vi "proba_2.vi"() -> ()   [LabVIEW 2015]
uses:
  <vilib>/MakerHub/LINX/Public/Peripherals/Digital/Digital Write N Chans.vi
  <vilib>/MakerHub/LINX/Public/Peripherals/Analog/Analog Read 1 Chan.vi
  <vilib>/MakerHub/LINX/Private/Local IO/LinxDigitalWrite.vi
  <vilib>/MakerHub/LINX/Public/Utilities/Check Channel.vi
  <vilib>/MakerHub/LINX/Public/Peripherals/Analog/Analog Read N Chans.vi
  <vilib>/MakerHub/LINX/Private/Local IO/LinxAnalogRead.vi
  <vilib>/MakerHub/LINX/Public/Utilities/Open Serial.vi
  <vilib>/MakerHub/LINX/Private/Utilties/Generate Error.vi
  <vilib>/MakerHub/LINX/LMH-LINX.lvlib
panel:
  out "x-y":u32
  out "appended array":bool[](array[boolean])
  in  "Stop Button":bool
  in  "Sample_1 (time)":dbl[][](array[numeric])
  in  "stop":bool
  in  "Sample_2 (time)":dbl[][](array[numeric])
  in  "Sample_3 (time)":dbl[][](array[numeric])
  in  "Sample_4 (time)":dbl[][](array[numeric])
  in  "LED_5 (time)":dbl[][](array[numeric])
  in  "Temp/Gap_1 (time)":dbl[][](array[numeric])
  in  "Temp/Gap_2 (time)":dbl[][](array[numeric])
  in  "Temp/Gap_3 (time)":dbl[][](array[numeric])
  in  "Temp/Gap_4 (time) 2":dbl[][](array[numeric])
  out "Ref":dbl(graph)
  in  "LED":refnum<visa-resource-name>="N/A"
  out "3":dbl(graph)
  out "2":dbl(graph)
  out "4":dbl(graph)
  out "1":dbl(graph)
  in  "milliseconds to wait":u32
  in  "Serial Port Analog":refnum<visa-resource-name>="N/A"
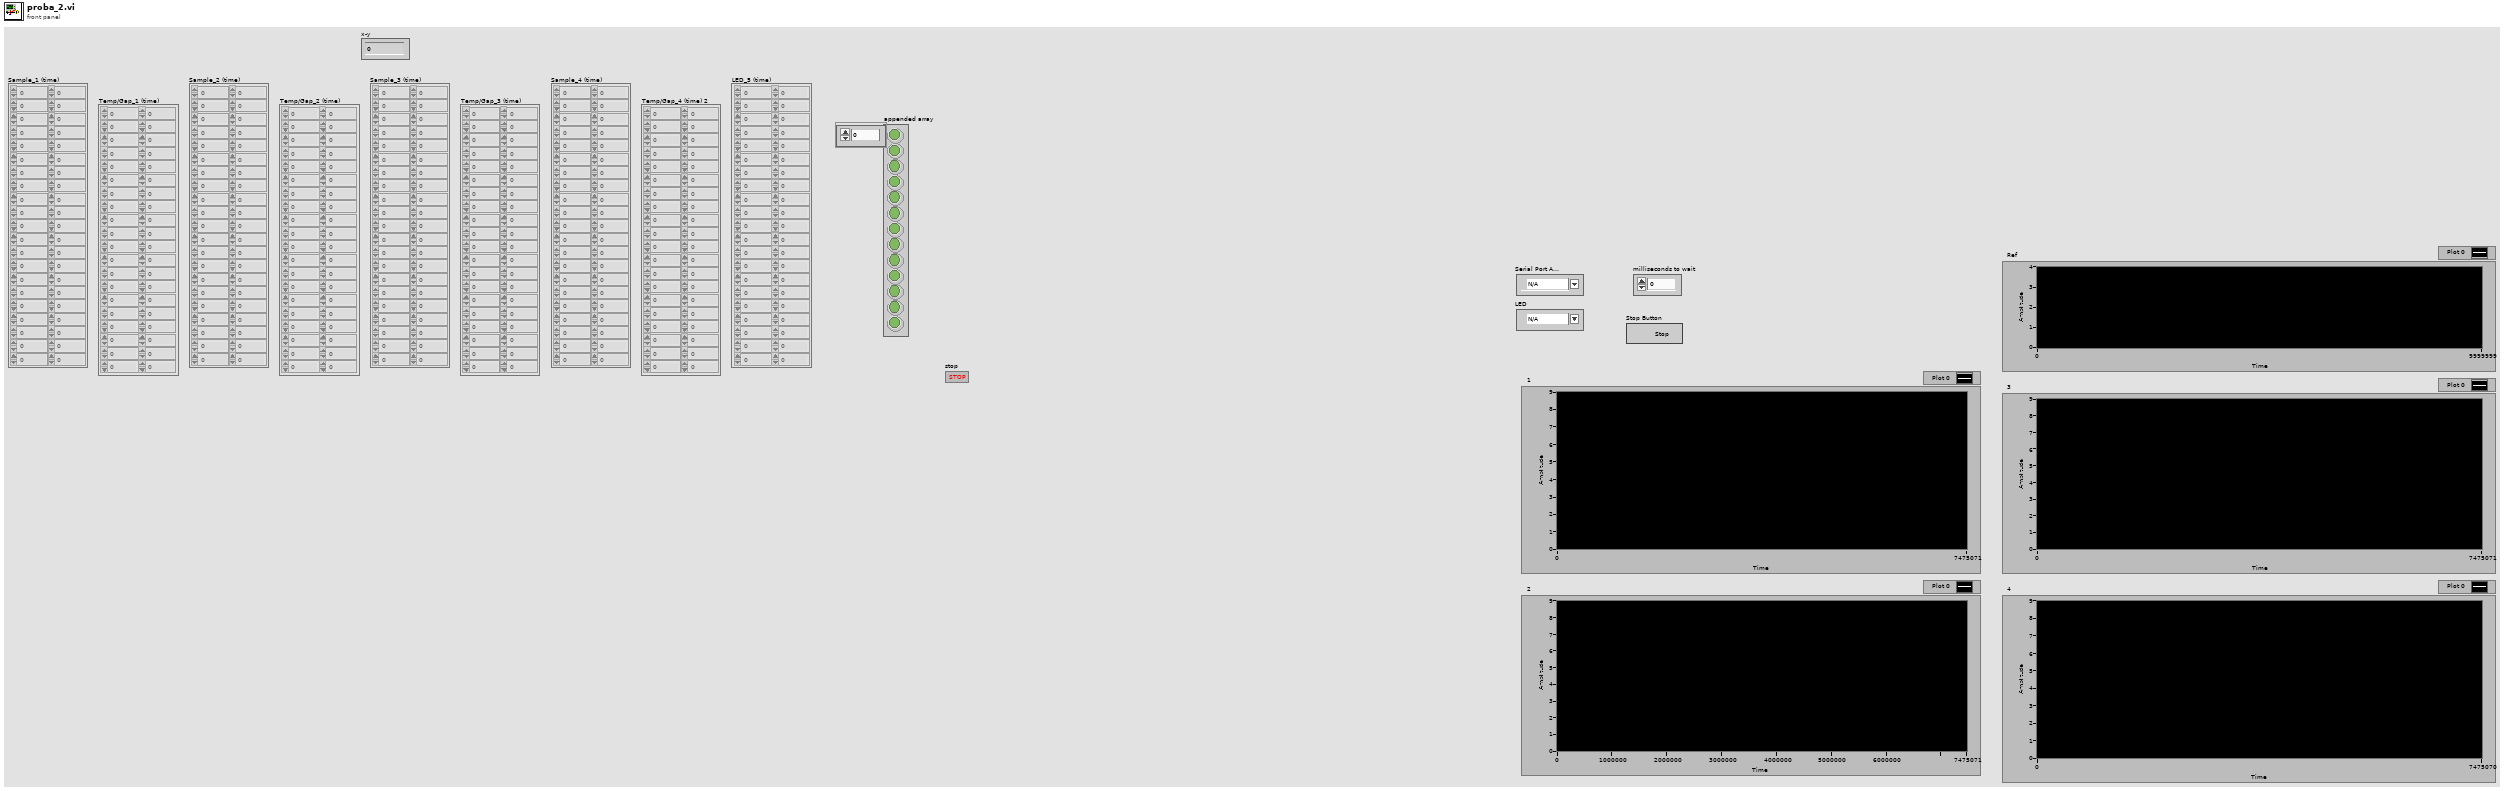
[diagram p1: front panel]
types:
  T1 = enum16{"open", "replace", "create", "open or create", "replace or create", "replace or create with confirmation"}
  T2 = typedef "LMH-LINX.lvlib/LINX Ref.ctl" = cluster{"IO":T3, "Interface":T4, "LINX Device Config":T5}
  T3 = typedef "LMH-LINX.lvlib/Platform.ctl" = enum16{"Remote", "Local"}
  T4 = typedef "LMH-LINX.lvlib/Interface.ctl" = enum16{"Serial", "TCP"}
  T5 = typedef "LMH-LINX.lvlib/Device.lvlib/LINX Device Config.ctl" = cluster{"Interface":T4, "COM Port":refnum<visa-resource-name>, "TCP Configuration":T6, "Device Family":u8, "Device ID":u8, "Device Name":string, "TCP Ref":refnum<k5>, "Channels":T7}
  T6 = typedef "LMH-LINX.lvlib/Device.lvlib/TCP Config.ctl" = cluster{"IP Address":string, "Port":u16}
  T7 = typedef "LMH-LINX.lvlib/Channels.ctl" = cluster{"DI":u8[], "DO":u8[], "AI":u8[], "AO":u8[], "PWM":u8[], "QE":u8[], "UART":u8[], "I2C 2":u8[], "SPI":u8[], "CAN":u8[], "Servo":u8[], "AI Ref (V)":dbl, "AI Resolution (Bits)":u8, "AO Ref (V)":dbl, "AO Resolution (Bits)":u8}
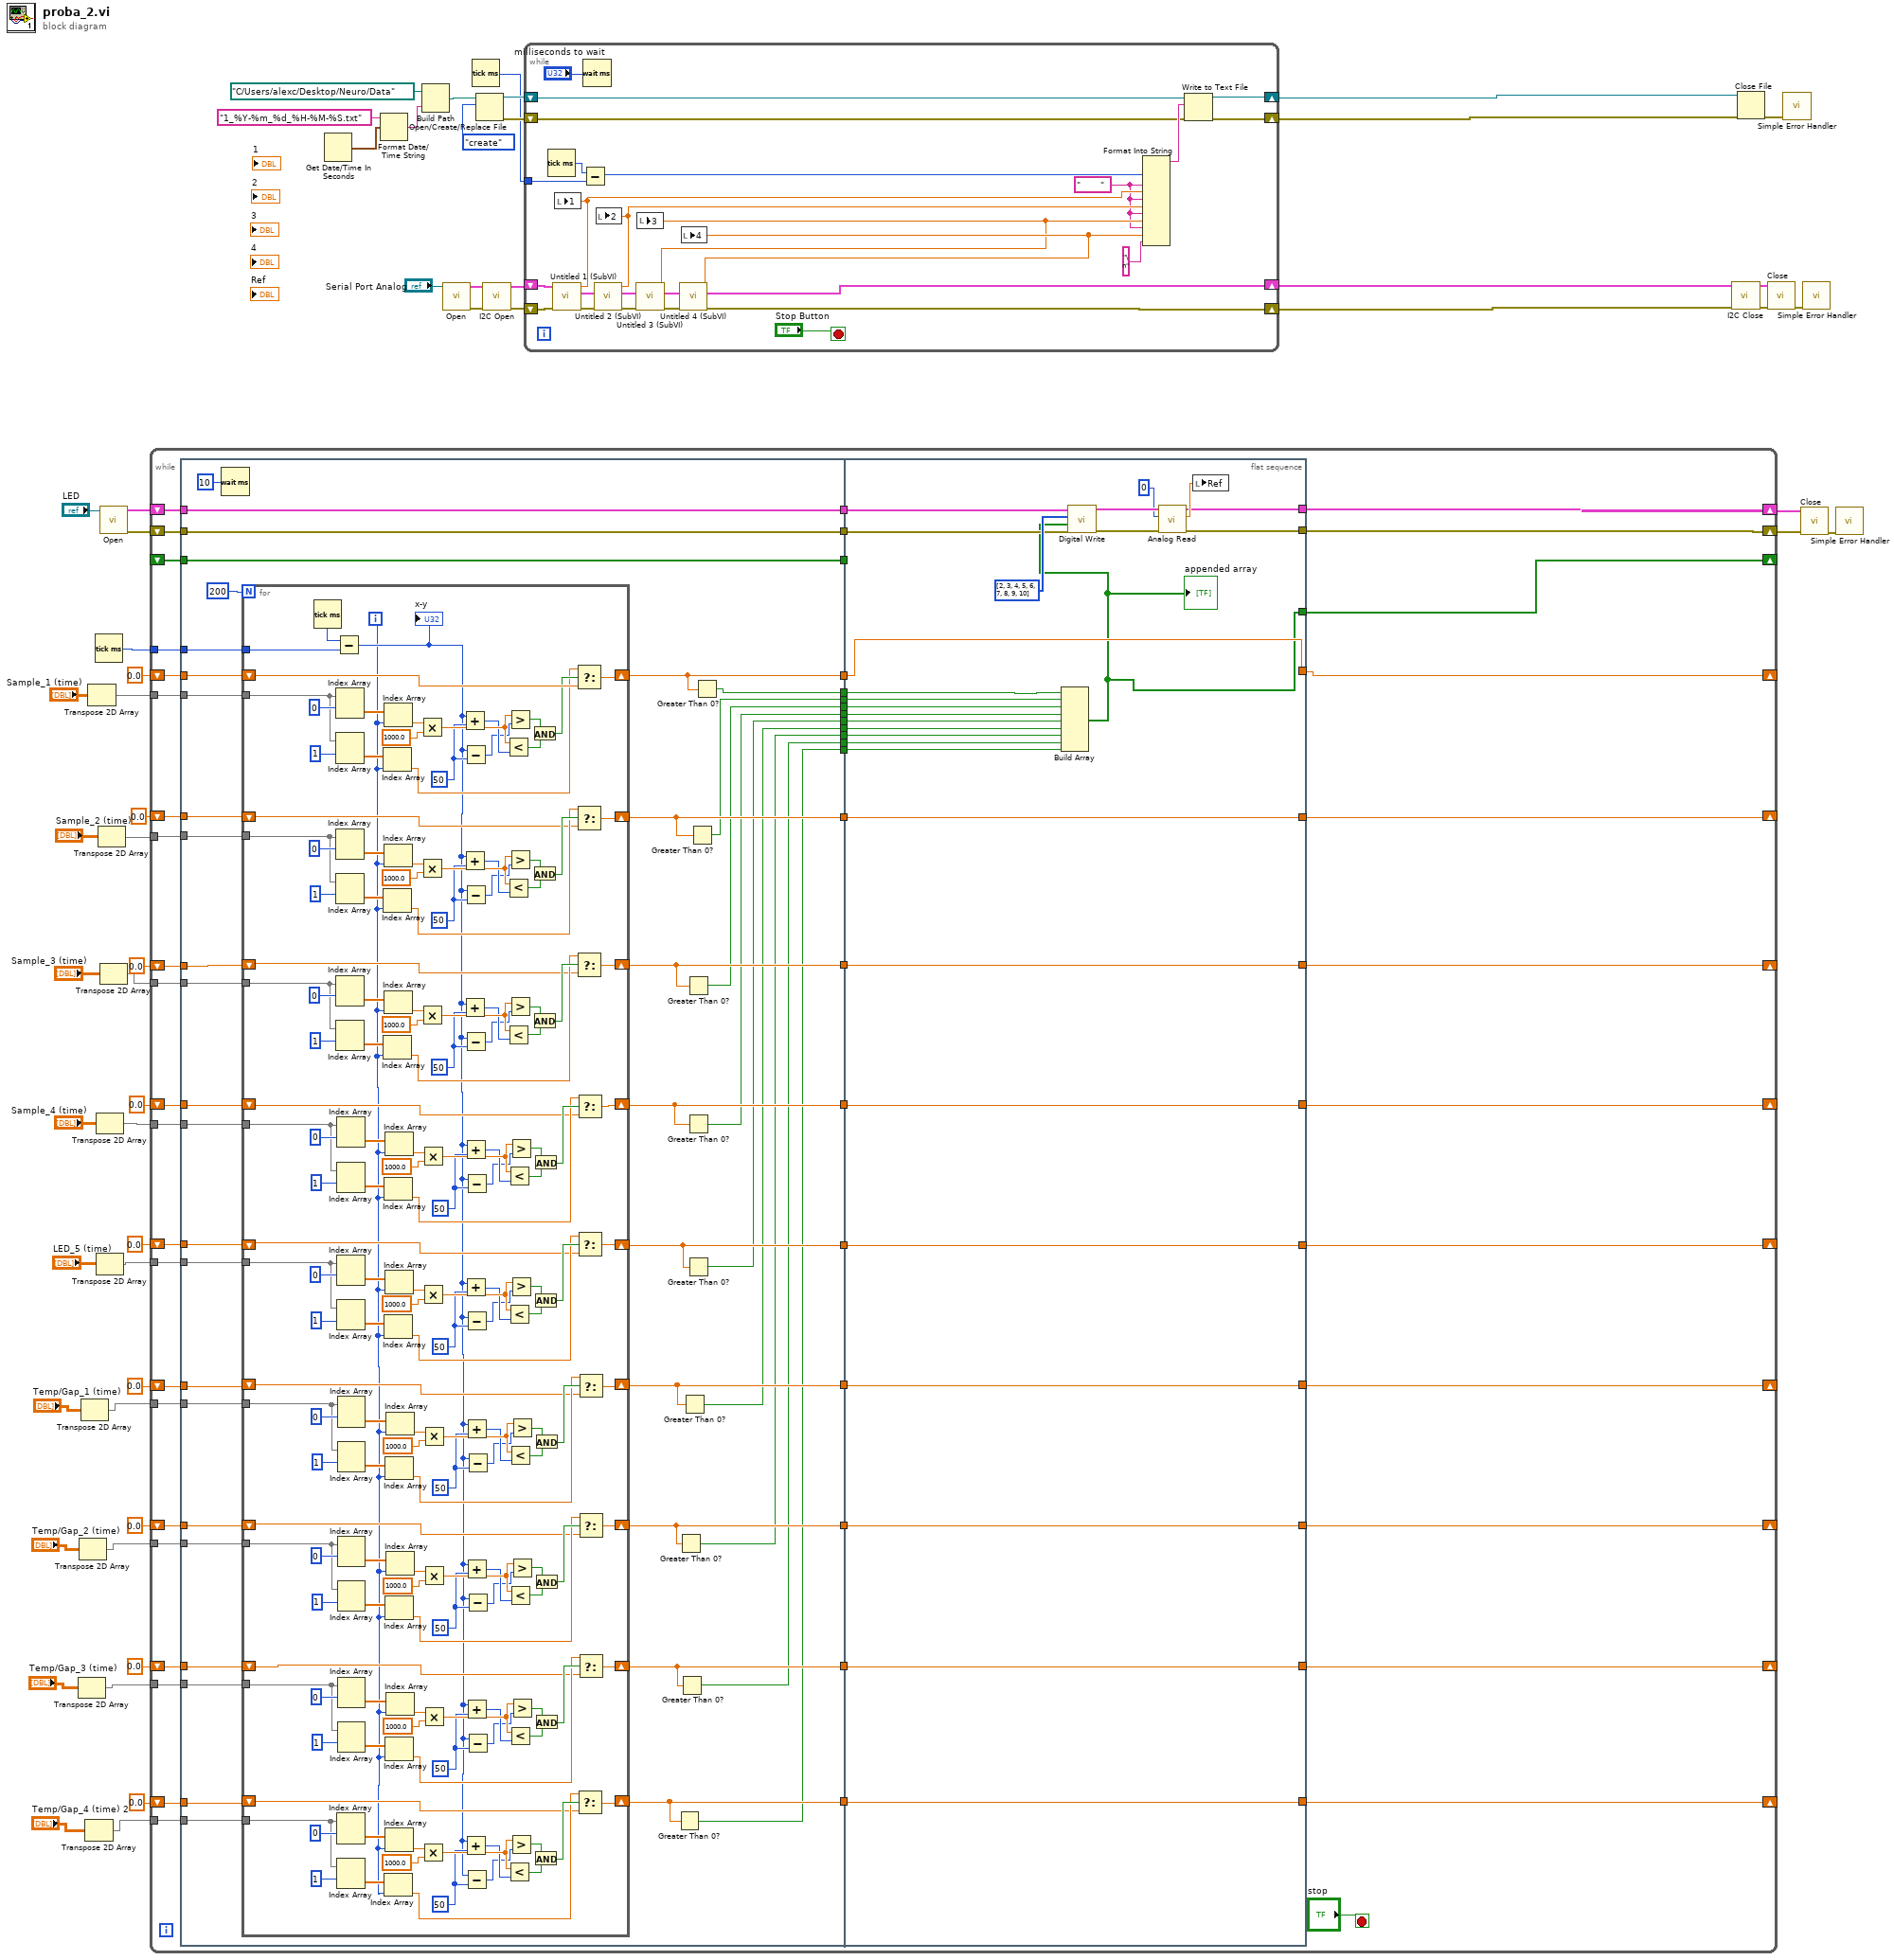
[diagram p0: block diagram]
diagram:
  n1 = Transpose 2D Array(2D array="Temp/Gap_3 (time)") -> (transposed array=w11:dbl[][])
  n2 = Transpose 2D Array(2D array="Temp/Gap_2 (time)") -> (transposed array=w12:dbl[][])
  n3 = Transpose 2D Array(2D array="Temp/Gap_1 (time)") -> (transposed array=w13:dbl[][])
  n4 = Transpose 2D Array(2D array="Temp/Gap_4 (time) 2") -> (transposed array=w10:dbl[][])
  n5 = Transpose 2D Array(2D array="Sample_1 (time)") -> (transposed array=w26:dbl[][])
  n6 = Tick Count (ms)() -> (millisecond timer value=w30:u32)
  n7 = Transpose 2D Array(2D array="Sample_4 (time)") -> (transposed array=w15:dbl[][])
  n8 = Transpose 2D Array(2D array="LED_5 (time)") -> (transposed array=w14:dbl[][])
  n9 = Transpose 2D Array(2D array="Sample_2 (time)") -> (transposed array=w24:dbl[][])
  n10 = call-poly <vilib>:"Open.vi"("Serial Port"="LED") -> ("Error Out"=w31:errorcluster, "LINX Resource"=w32:T2)  [unwired: 8 in, 1 out]
  n11 = Transpose 2D Array(2D array="Sample_3 (time)") -> (transposed array=w16:dbl[][])
  n12 = while {
    tunnel: w30 -> [w110]
    shift-right: [w60] -> _
    shift-left: 0.0 ("Numeric") -> [w112]
    shift-right: [w66] -> w29
    shift-left: w32 -> [w63]
    shift-right: [w65] -> w28
    shift-left: w31 -> [w61]
    tunnel: w26 -> [w109]
    tunnel: w24 -> [w108]
    shift-right: [w85] -> _
    shift-left: 0.0 ("Numeric") -> [w107]
    tunnel: w11 -> [w106]
    tunnel: w16 -> [w105]
    tunnel: w15 -> [w104]
    tunnel: w14 -> [w103]
    tunnel: w13 -> [w102]
    tunnel: w12 -> [w101]
    tunnel: w10 -> [w100]
    shift-right: [w86] -> _
    shift-left: 0.0 ("Numeric") -> [w99]
    shift-right: [w87] -> _
    shift-left: 0.0 ("Numeric") -> [w98]
    shift-right: [w88] -> _
    shift-left: 0.0 ("Numeric") -> [w97]
    shift-right: [w90] -> _
    shift-left: 0.0 ("Numeric") -> [w96]
    shift-right: [w91] -> _
    shift-left: 0.0 ("Numeric") -> [w95]
    shift-right: [w92] -> _
    shift-left: 0.0 ("Numeric") -> [w94]
    shift-right: [w89] -> _
    shift-left: 0.0 ("Numeric") -> [w93]
    shift-right: [w59] -> _
    shift-left: _ -> [w58]
    stop <- "stop" stop-if-true
    n13 = flat-sequence {
      tunnel: w112 -> [w154]
      tunnel: w110 -> [w153]
      tunnel: w109 -> [w152]
      tunnel: w108 -> [w149]
      tunnel: w107 -> [w148]
      tunnel: w106 -> [w147]
      tunnel: w105 -> [w146]
      tunnel: w104 -> [w145]
      tunnel: w103 -> [w144]
      tunnel: w102 -> [w143]
      tunnel: w101 -> [w142]
      tunnel: w100 -> [w141]
      tunnel: w99 -> [w140]
      tunnel: w98 -> [w139]
      tunnel: w97 -> [w138]
      tunnel: w96 -> [w137]
      tunnel: w95 -> [w136]
      tunnel: w94 -> [w135]
      tunnel: w93 -> [w134]
      tunnel: [w133] -> w84
      tunnel: [w132] -> w83
      tunnel: [w131] -> w82
      tunnel: [w130] -> w81
      tunnel: [w129] -> w80
      tunnel: [w128] -> w79
      tunnel: [w127] -> w78
      tunnel: [w126] -> w77
      tunnel: [w125] -> w76
      tunnel: [w124] -> w75
      tunnel: [w123] -> w74
      tunnel: [w122] -> w73
      tunnel: [w121] -> w72
      tunnel: [w120] -> w71
      tunnel: [w119] -> w70
      tunnel: [w118] -> w69
      tunnel: [w117] -> w68
      tunnel: [w116] -> w67
      tunnel: [w115] -> w64
      tunnel: w63 -> [w115]
      tunnel: [w114] -> w62
      tunnel: w61 -> [w114]
      tunnel: w58 -> [w113]
      tunnel: [w113] -> w57
      tunnel: [w332] -> w85
      tunnel: [w333] -> w86
      tunnel: [w334] -> w87
      tunnel: [w335] -> w88
      tunnel: [w336] -> w89
      tunnel: [w337] -> w90
      tunnel: [w338] -> w91
      tunnel: [w339] -> w92
      tunnel: w84 -> [w339]
      tunnel: w83 -> [w338]
      tunnel: w82 -> [w337]
      tunnel: w81 -> [w336]
      tunnel: w80 -> [w335]
      tunnel: w79 -> [w334]
      tunnel: w78 -> [w333]
      tunnel: w77 -> [w332]
      tunnel: w76 -> [w326]
      tunnel: w75 -> [w322]
      tunnel: w74 -> [w321]
      tunnel: w73 -> [w320]
      tunnel: w72 -> [w319]
      tunnel: w71 -> [w318]
      tunnel: w70 -> [w317]
      tunnel: w69 -> [w316]
      tunnel: w68 -> [w315]
      tunnel: w67 -> [w325]
      tunnel: [w326] -> w60
      tunnel: [w324] -> w66
      tunnel: [w323] -> w65
      tunnel: w64 -> [w314]
      tunnel: w62 -> [w313]
      tunnel: [w312] -> w59
      tunnel: w57 -> [_]
      frame #0 {
        n14 = Wait (ms)(milliseconds to wait=u32 10) -> ()  [unwired: 1 out]
        n15 = for {
          N: 200 -> [_]
          tunnel: w153 -> [w311]
          shift-right: [w310] -> w125
          shift-left: w154 -> [w309]
          tunnel: w152 -> [w303]
          shift-right: [w278] -> w126
          shift-left: w148 -> [w277]
          tunnel: w149 -> [w276]
          shift-right: [w247] -> w127
          shift-left: w140 -> [w246]
          shift-right: [w245] -> w128
          shift-left: w139 -> [w244]
          shift-right: [w173] -> w129
          shift-left: w138 -> [w172]
          shift-right: [w170] -> w131
          shift-left: w137 -> [w171]
          shift-right: [w169] -> w132
          shift-left: w136 -> [w168]
          shift-right: [w166] -> w133
          shift-left: w135 -> [w167]
          shift-right: [w164] -> w130
          shift-left: w134 -> [w165]
          tunnel: w147 -> [w162]
          tunnel: w146 -> [w161]
          tunnel: w145 -> [w160]
          tunnel: w144 -> [w159]
          tunnel: w143 -> [w158]
          tunnel: w142 -> [w157]
          tunnel: w141 -> [w156]
          i -> [w155]
          w178 = u32 50 ("y")
          w192 = u32 50 ("y")
          w206 = u32 50 ("y")
          w220 = u32 50 ("y")
          w234 = u32 50 ("y")
          w252 = u32 50 ("y")
          w266 = u32 50 ("y")
          w283 = u32 50 ("y")
          w297 = u32 50 ("y")
          n16 = Tick Count (ms)() -> (millisecond timer value=w308:u32)
          n17 = Subtract(x=w308, y=w311) -> (x-y=w163:u32)
          "x-y" <- w163
          n18 = Index Array(array=w303, index (row)=0) -> (element=w305:dbl[])  [unwired: 1 in]
          n19 = Index Array(array=w303, index (row)=1) -> (element=w304:dbl[])  [unwired: 1 in]
          n20 = Index Array(array=w276, index (row)=0) -> (element=w290:dbl[])  [unwired: 1 in]
          n21 = Index Array(array=w276, index (row)=1) -> (element=w289:dbl[])  [unwired: 1 in]
          n22 = Index Array(array=w161, index (row)=0) -> (element=w273:dbl[])  [unwired: 1 in]
          n23 = Index Array(array=w161, index (row)=1) -> (element=w272:dbl[])  [unwired: 1 in]
          n24 = Index Array(array=w160, index (row)=0) -> (element=w259:dbl[])  [unwired: 1 in]
          n25 = Index Array(array=w160, index (row)=1) -> (element=w258:dbl[])  [unwired: 1 in]
          n26 = Index Array(array=w159, index (row)=0) -> (element=w241:dbl[])  [unwired: 1 in]
          n27 = Index Array(array=w159, index (row)=1) -> (element=w240:dbl[])  [unwired: 1 in]
          n28 = Index Array(array=w156, index (row)=0) -> (element=w185:dbl[])  [unwired: 1 in]
          n29 = Index Array(array=w156, index (row)=1) -> (element=w184:dbl[])  [unwired: 1 in]
          n30 = Index Array(array=w158, index (row)=0) -> (element=w227:dbl[])  [unwired: 1 in]
          n31 = Index Array(array=w158, index (row)=1) -> (element=w226:dbl[])  [unwired: 1 in]
          n32 = Index Array(array=w157, index (row)=0) -> (element=w213:dbl[])  [unwired: 1 in]
          n33 = Index Array(array=w157, index (row)=1) -> (element=w212:dbl[])  [unwired: 1 in]
          n34 = Index Array(array=w162, index (row)=0) -> (element=w199:dbl[])  [unwired: 1 in]
          n35 = Index Array(array=w162, index (row)=1) -> (element=w198:dbl[])  [unwired: 1 in]
          n36 = Index Array(array=w304, index=w155) -> (element=w293:dbl)
          n37 = Index Array(array=w289, index=w155) -> (element=w279:dbl)
          n38 = Index Array(array=w272, index=w155) -> (element=w262:dbl)
          n39 = Index Array(array=w305, index=w155) -> (element=w302:dbl)
          n40 = Index Array(array=w290, index=w155) -> (element=w288:dbl)
          n41 = Index Array(array=w273, index=w155) -> (element=w271:dbl)
          n42 = Index Array(array=w258, index=w155) -> (element=w248:dbl)
          n43 = Index Array(array=w240, index=w155) -> (element=w230:dbl)
          n44 = Index Array(array=w184, index=w155) -> (element=w174:dbl)
          n45 = Index Array(array=w259, index=w155) -> (element=w257:dbl)
          n46 = Index Array(array=w241, index=w155) -> (element=w239:dbl)
          n47 = Index Array(array=w226, index=w155) -> (element=w216:dbl)
          n48 = Index Array(array=w212, index=w155) -> (element=w202:dbl)
          n49 = Index Array(array=w198, index=w155) -> (element=w188:dbl)
          n50 = Index Array(array=w185, index=w155) -> (element=w183:dbl)
          n51 = Index Array(array=w227, index=w155) -> (element=w225:dbl)
          n52 = Index Array(array=w213, index=w155) -> (element=w211:dbl)
          n53 = Index Array(array=w199, index=w155) -> (element=w197:dbl)
          n54 = Multiply(x=w302, y=1000.0) -> (x*y=w298:dbl)
          n55 = Multiply(x=w288, y=1000.0) -> (x*y=w284:dbl)
          n56 = Multiply(x=w271, y=1000.0) -> (x*y=w267:dbl)
          n57 = Multiply(x=w257, y=1000.0) -> (x*y=w253:dbl)
          n58 = Multiply(x=w239, y=1000.0) -> (x*y=w235:dbl)
          n59 = Multiply(x=w183, y=1000.0) -> (x*y=w179:dbl)
          n60 = Multiply(x=w225, y=1000.0) -> (x*y=w221:dbl)
          n61 = Multiply(x=w211, y=1000.0) -> (x*y=w207:dbl)
          n62 = Multiply(x=w197, y=1000.0) -> (x*y=w193:dbl)
          n63 = Add(x=w163, y=w297) -> (x+y=w296:u32)
          n64 = Add(x=w163, y=w283) -> (x+y=w282:u32)
          n65 = Add(x=w163, y=w266) -> (x+y=w265:u32)
          n66 = Subtract(x=w163, y=w297) -> (x-y=w295:u32)
          n67 = Subtract(x=w163, y=w283) -> (x-y=w281:u32)
          n68 = Subtract(x=w163, y=w266) -> (x-y=w264:u32)
          n69 = Add(x=w163, y=w252) -> (x+y=w251:u32)
          n70 = Add(x=w163, y=w234) -> (x+y=w233:u32)
          n71 = Add(x=w163, y=w178) -> (x+y=w177:u32)
          n72 = Subtract(x=w163, y=w252) -> (x-y=w250:u32)
          n73 = Subtract(x=w163, y=w234) -> (x-y=w232:u32)
          n74 = Add(x=w163, y=w220) -> (x+y=w219:u32)
          n75 = Add(x=w163, y=w206) -> (x+y=w205:u32)
          n76 = Add(x=w163, y=w192) -> (x+y=w191:u32)
          n77 = Subtract(x=w163, y=w178) -> (x-y=w176:u32)
          n78 = Subtract(x=w163, y=w220) -> (x-y=w218:u32)
          n79 = Subtract(x=w163, y=w206) -> (x-y=w204:u32)
          n80 = Subtract(x=w163, y=w192) -> (x-y=w190:u32)
          n81 = Less?(x=w298, y=w296) -> (x < y?=w300:bool)
          n82 = Less?(x=w284, y=w282) -> (x < y?=w286:bool)
          n83 = Less?(x=w267, y=w265) -> (x < y?=w269:bool)
          n84 = Less?(x=w253, y=w251) -> (x < y?=w255:bool)
          n85 = Less?(x=w235, y=w233) -> (x < y?=w237:bool)
          n86 = Less?(x=w179, y=w177) -> (x < y?=w181:bool)
          n87 = Greater?(x=w298, y=w295) -> (0:w301:bool)
          n88 = Greater?(x=w284, y=w281) -> (0:w287:bool)
          n89 = Greater?(x=w267, y=w264) -> (0:w270:bool)
          n90 = Less?(x=w221, y=w219) -> (x < y?=w223:bool)
          n91 = Less?(x=w207, y=w205) -> (x < y?=w209:bool)
          n92 = Less?(x=w193, y=w191) -> (x < y?=w195:bool)
          n93 = Greater?(x=w253, y=w250) -> (0:w256:bool)
          n94 = Greater?(x=w235, y=w232) -> (0:w238:bool)
          n95 = Greater?(x=w179, y=w176) -> (0:w182:bool)
          n96 = Greater?(x=w221, y=w218) -> (0:w224:bool)
          n97 = Greater?(x=w207, y=w204) -> (0:w210:bool)
          n98 = Greater?(x=w193, y=w190) -> (0:w196:bool)
          n99 = And(x=w301, y=w300) -> (x .and. y?=w294:bool)
          n100 = And(x=w287, y=w286) -> (x .and. y?=w280:bool)
          n101 = And(x=w270, y=w269) -> (x .and. y?=w263:bool)
          n102 = And(x=w256, y=w255) -> (x .and. y?=w249:bool)
          n103 = And(x=w238, y=w237) -> (x .and. y?=w231:bool)
          n104 = And(x=w182, y=w181) -> (x .and. y?=w175:bool)
          n105 = And(x=w224, y=w223) -> (x .and. y?=w217:bool)
          n106 = And(x=w210, y=w209) -> (x .and. y?=w203:bool)
          n107 = And(x=w196, y=w195) -> (x .and. y?=w189:bool)
          n108 = Select(t=w293, s=w294, f=w309) -> (s? t:f=w310:dbl)
          n109 = Select(t=w279, s=w280, f=w277) -> (s? t:f=w278:dbl)
          n110 = Select(t=w262, s=w263, f=w246) -> (s? t:f=w247:dbl)
          n111 = Select(t=w248, s=w249, f=w244) -> (s? t:f=w245:dbl)
          n112 = Select(t=w230, s=w231, f=w172) -> (s? t:f=w173:dbl)
          n113 = Select(t=w174, s=w175, f=w165) -> (s? t:f=w164:dbl)
          n114 = Select(t=w216, s=w217, f=w171) -> (s? t:f=w170:dbl)
          n115 = Select(t=w202, s=w203, f=w168) -> (s? t:f=w169:dbl)
          n116 = Select(t=w188, s=w189, f=w167) -> (s? t:f=w166:dbl)
        }
        n117 = Greater Than 0?(x=w130) -> (x > 0?=w117:bool)
        n118 = Greater Than 0?(x=w132) -> (x > 0?=w119:bool)
        n119 = Greater Than 0?(x=w133) -> (x > 0?=w118:bool)
        n120 = Greater Than 0?(x=w131) -> (x > 0?=w120:bool)
        n121 = Greater Than 0?(x=w127) -> (x > 0?=w123:bool)
        n122 = Greater Than 0?(x=w128) -> (x > 0?=w122:bool)
        n123 = Greater Than 0?(x=w129) -> (x > 0?=w121:bool)
        n124 = Greater Than 0?(x=w126) -> (x > 0?=w124:bool)
        n125 = Greater Than 0?(x=w125) -> (x > 0?=w116:bool)
      }
      frame #1 {
        n126 = Build Array(w325, w322, w321, w320, w319, w318, w317, w316, w315) -> (w312:bool[])
        "appended array" <- w312
        n127 = call-poly <vilib>:"Digital Write.vi"("Error In"=w313, "Values"=w312, "DO Channels"=u8[] [2, 3, 4, 5, 6, 7, 8, 9, 10], "LINX Resource"=w314) -> ("Error Out"=w331:errorcluster, "LINX Resource"=w330:T2)  [unwired: 6 in]
        n128 = call-poly <vilib>:"Analog Read.vi"("Error In"=w331, "Analog Channel"=u8 0, "LINX Resource"=w330) -> ("Error Out"=w323:errorcluster, "Voltage"=w327:dbl, "LINX Resource"=w324:T2)  [unwired: 5 in, 1 out]
        n129 = local write "Ref"(w327) -> ()
      }
    }
  }
  n130 = Get Date/Time In Seconds() -> (seconds since 1Jan1904=w49:timestamp)
  n131 = Format Date/Time String(time format string (%c)="1_%Y-%m_%d_%H-%M-%S.txt", seconds (now)=w49) -> (date/time string=w51:string)  [unwired: 1 in]
  n132 = Build Path(base path=path "C:/Users/alexc/Desktop/Neuro/Data", name or relative path=w51) -> (appended path=w48:path)
  n133 = call-poly <vilib>:"Open.vi"("Serial Port"="Serial Port Analog") -> ("Error Out"=w55:errorcluster, "LINX Resource"=w56:T2)  [unwired: 8 in, 1 out]
  n134 = Tick Count (ms)() -> (millisecond timer value=w44:u32)
  n135 = Open/Create/Replace File(file path (use dialog)=w48, operation (0:open)=T1."create") -> (refnum out=w46:refnum<file>, error out=w45:errorcluster)  [unwired: 4 in, 1 out]
  n136 = call <vilib>:"I2C Open.vi"("Error In"=w55, "LINX Resource"=w56) -> ("Error Out"=w42:errorcluster, "LINX Resource"=w43:T2)  [unwired: 8 in]
  n137 = while {
    tunnel: w44 -> [w358]
    shift-right: [w354] -> w34
    shift-left: w46 -> [w356]
    shift-right: [w353] -> w33
    shift-left: w45 -> [w355]
    shift-right: [w350] -> w36
    shift-left: w43 -> [w352]
    shift-right: [w349] -> w35
    shift-left: w42 -> [w351]
    stop <- "Stop Button" stop-if-true
    w343 = "       "
    n138 = Tick Count (ms)() -> (millisecond timer value=w359:u32)
    n139 = call "Untitled 1 (SubVI).vi"("error in (no error)"=w351, "LINX Resource in"=w352) -> ("error out"=w364:errorcluster, "LINX Resource out"=w365:T2, "Numeric"=w347:dbl)  [unwired: 7 in]
    n140 = local write "1"(w347) -> ()
    n141 = Subtract(x=w359, y=w358) -> (x-y=w344:u32)
    n142 = Wait (ms)(milliseconds to wait="milliseconds to wait") -> ()  [unwired: 1 out]
    n143 = call "Untitled 2 (SubVI).vi"("error in (no error)"=w364, "LINX Resource in"=w365) -> ("error out"=w363:errorcluster, "LINX Resource"=w362:T2, "Numeric"=w346:dbl)  [unwired: 7 in]
    n144 = local write "2"(w346) -> ()
    n145 = call "Untitled 3 (SubVI).vi"("error in (no error)"=w363, "LINX Resource in"=w362) -> ("error out"=w360:errorcluster, "LINX Resource out"=w361:T2, "Numeric"=w345:dbl)  [unwired: 7 in]
    n146 = local write "3"(w345) -> ()
    n147 = call "Untitled 4 (SubVI).vi"("error in (no error)"=w360, "LINX Resource in"=w361) -> ("error out"=w349:errorcluster, "LINX Resource"=w350:T2, "Numeric"=w348:dbl)  [unwired: 7 in]
    n148 = local write "4"(w348) -> ()
    n149 = Format Into String(w344, w343, w347, w343, w346, w343, w345, w343, w348, "\n" ("input 10")) -> (resulting string=w357:string)  [unwired: 3 in, 1 out]
    n150 = Write to Text File(file (use dialog)=w356, text=w357, error in=w355) -> (refnum out=w354:refnum<file>, error out=w353:errorcluster)  [unwired: 1 in, 1 out]
  }
  n151 = call <vilib>:"I2C Close.vi"("Error In"=w35, "LINX Resource"=w36) -> ("Error Out"=w38:errorcluster, "LINX Resource"=w39:T2)  [unwired: 8 in]
  n152 = Close File(refnum=w34, error in=w33) -> (error out=w41:errorcluster)  [unwired: 1 out]
  n153 = call <vilib>:"Close.vi"("Error In"=w38, "LINX Resource"=w39) -> ("Error Out"=w40:errorcluster)  [unwired: 9 in]
  n154 = call <vilib>:"Simple Error Handler.vi"("error in (no error)"=w41) -> ()  [unwired: 4 in, 5 out]
  n155 = call <vilib>:"Close.vi"("Error In"=w28, "LINX Resource"=w29) -> ("Error Out"=w37:errorcluster)  [unwired: 9 in]
  n156 = call <vilib>:"Simple Error Handler.vi"("error in (no error)"=w40) -> ()  [unwired: 4 in, 5 out]
  n157 = call <vilib>:"Simple Error Handler.vi"("error in (no error)"=w37) -> ()  [unwired: 4 in, 5 out]
